vi "select standards.vi"(0 "standards array":T5=[{"Standard Description"="Nitrate (molar)", "standards setup"={"integration time"=0.0, "rinse time"=0.0, "sample time"=0.0, "sample type"=0}, "Standard C"=[0.0, 1e-05, 3e-05, 0.0001, 0.0003, 0.001], "extinction"=array[316 elements], "Your name"="Monroe Weber-Shirk", "correlation coef"=[], "units"=""}, {"Standard Description"="Methylene Blue (molar)", "standards setup"={"integration time"=0.0, "rinse time"=0.0, "sample time"=0.0, "sample type"=0}, "Standard C"=[0.0, 1e-05, 3e-05, 0.0001, 0.0003, 0.001], "extinction"=array[316 elements], "Your name"="Monroe Weber-Shirk", "correlation coef"=[], "units"=""}, {"Standard Description"="Nitrate (molar)", "standards setup"={"integration time"=0.0, "rinse time"=0.0, "sample time"=0.0, "sample type"=0}, "Standard C"=[0.0, 1e-05, 3e-05, 0.0001, 0.0003, 0.001], "extinction"=[6e-05, 0.00221, 0.00306, 0.00317, 0.00265, 0.00207, 0.00119, 0.00025, -0.00096, -0.00199, -0.00326, -0.00411, -0.00514, -0.00601, -0.00637, -0.00648, -0.00656, -0.00639, -0.00598, -0.00572, -0.00506, -0.00451, -0.00396, -0.0035, -0.00303, -0.00267, -0.00244, -0.00225, -0.00195, -0.00143, -0.00079, 3e-05, 0.0008, 0.00166, 0.00238, 0.00297, 0.00341, 0.00378, 0.0039, 0.00392, 0.00384, 0.00372, 0.00352, 0.00314, 0.00282, 0.00242, 0.00177, 0.00137, 0.00077, -1e-05, -0.00059, -0.00108, -0.00134, -0.00131, -0.00105, -0.00088, -0.00057, -0.00032, -0.00022, -0.00033, -0.00038, -0.00019, -0.00021, -0.00013, -0.00021, -0.00012, -0.00018, -6e-05, -0.00015, -0.00013, -7e-05, -1e-05, 4e-05, 0.00028, 0.00035, 0.00048, 0.00077, 0.0008, 0.00097, 0.00123, 0.00125, 0.00146, 0.00151, 0.00158, 0.00175, 0.00189, 0.00192, 0.00209, 0.00259, 0.00344, 0.00344, 0.00314, 0.00273, 0.00338, 0.00329, 0.00483, 0.00416, 0.00453, 0.00415, 0.0057, 0.00456, 0.00387, 0.00733, 0.00433, 0.00578, 0.00793, 0.00433, 0.00503, 0.00907, 0.00512, 0.00527, 0.00619, 0.00883, 0.00532, 0.00614, 0.00546, 0.01057, 0.01022, 0.00575, 0.00856, 0.01062, 0.01115, 0.00621, 0.00558, 0.00915, 0.00848, 0.00535, 0.00787, 0.00842, 0.00877, 0.00704, 0.00596, 0.00531, 0.00262, 0.00599, 0.00656, 0.00518, 0.00746, 0.01216, 0.0121, 0.00685, 0.00506, 0.0082, 0.00939, 0.00521, 0.00415, 0.00613, 0.00923, 0.00846, 0.01092, 0.01307, 0.00959, 0.0108, 0.01184, 0.01274, 0.00772, 0.01136, 0.01332, 0.00874, 0.0079, 0.0115, 0.01463, 0.01071, 0.00805, 0.01184, 0.0133, 0.01077, 0.00883, 0.01077, 0.00929, 0.009, 0.00866, 0.00807, 0.00978, 0.01129, 0.00897, 0.00906, 0.0057, 0.01086, 0.01492, 0.0093, 0.00859, 0.01165, 0.01368, 0.01042, 0.00794, 0.0093, 0.00512, -0.00669, -0.0079, -0.00685, 0.00434, -0.00195, 0.00642, 0.00312, 0.00416, -0.00061, -0.00059, -0.0019, -0.00566, -0.00833, 0.00254, 0.0, -0.00189, 0.00862, 0.00765, 0.00112, -0.00064, 0.0028, 0.00683, 0.00155, -0.0003, 0.0054, 0.00462, -0.00639, 0.00265, 0.00604, -0.00057, -0.00447, 0.00471, -0.00041, -0.01329, -0.00877, -0.0001, 0.0025, -0.01448, -0.01643, -0.01341, -0.0164, -0.00784, 0.00132, -0.00469, -0.00727, -0.00599, -0.00289, -0.0079, -0.00978, -0.00033, -0.0065, -0.01058, 0.00389, 0.00607, -0.00247, 0.00625, 0.00309, 0.0075, 0.00675, 0.00238, 0.02153, 0.00531, 0.00671, 0.01777, 0.00942, 0.01489, 0.02458, 0.00833, 0.00894, 0.0129, 0.01617, 0.02844, 0.01483, 0.01608, 0.02296, 0.01797, 0.01881, 0.0142, 0.00575, 0.00914, 0.01087, 0.01379, 0.01463, 0.0223, 0.00849, 0.01046, 0.00225, 0.01255, 0.00628, 0.00013, -0.01025, -0.00317, -0.00169, -0.00013, 0.014, 0.00627, 0.02648, 0.01156, 0.01533, 0.0162, 0.012, 0.00538, 0.01255, -0.00395, -0.00947, -0.0081, -0.0059, -0.00109, 0.01068, 0.00973, 0.0028, 0.00073, 0.01567, 0.01887, 0.02369, 0.02372, 0.01115, 0.01058, 0.00817, 0.00433, 0.00431, 0.01495, -0.00257, 0.00178, -0.00054, 0.00404, 0.01396, 0.00617], "Your name"="Monroe Weber-Shirk", "correlation coef"=[], "units"=""}] {"correlation coef" format="%.3f"; "extinction" format="%.2e"; "Standard C" format="%^.2e"; "standards setup"."sample type" items=["Sample Cuvet", "Sipper Cell", "No Dialog"]; "standards setup"."sample time" min=0.0 max=100.0 step=1.0 format="%.1f"; "standards setup"."rinse time" min=0.0 max=100.0 step=1.0 format="%.1f"; "standards setup"."integration time" format="%.1f"}, 11 "standard cluster array in":T2 {"Absorbance" format="%.2e"; "Concentrations" format="%.3e"; "Setup"."sample type" items=["Sample Cuvet", "Sipper Cell", "No Dialog"]; "Setup"."sample time" min=0.0 max=100.0 step=1.0 format="%.1f"; "Setup"."rinse time" min=0.0 max=100.0 step=1.0 format="%.1f"; "Setup"."integration time" format="%.1f"}) -> (10 "mixture cluster":T1 {"H array" format="%.2f"}, 15 "standard cluster array out":T2 {"Absorbance" format="%.2e"; "Concentrations" format="%.3e"; "Setup"."sample type" items=["Sample Cuvet", "Sipper Cell", "No Dialog"]; "Setup"."sample time" min=0.0 max=100.0 step=1.0 format="%.1f"; "Setup"."rinse time" min=0.0 max=100.0 step=1.0 format="%.1f"; "Setup"."integration time" format="%.1f"})   [LabVIEW 2015]
uses:
  standards array.ctl
  settings.ctl
  standard cluster array.ctl
  standard cluster.ctl
  mixture cluster.ctl
panel:
  in  "empty standard cluster array":T2 {"Absorbance" format="%.2e"; "Concentrations" format="%.3e"; "Setup"."sample type" items=["Sample Cuvet", "Sipper Cell", "No Dialog"]; "Setup"."sample time" min=0.0 max=100.0 step=1.0 format="%.1f"; "Setup"."rinse time" min=0.0 max=100.0 step=1.0 format="%.1f"; "Setup"."integration time" format="%.1f"}
  in  "empty array":T5 {"correlation coef" format="%.3f"; "extinction" format="%.2e"; "Standard C" format="%^.2e"; "standards setup"."sample type" items=["Sample Cuvet", "Sipper Cell", "No Dialog"]; "standards setup"."sample time" min=0.0 max=100.0 step=1.0 format="%.1f"; "standards setup"."rinse time" min=0.0 max=100.0 step=1.0 format="%.1f"; "standards setup"."integration time" format="%.1f"}
  in  "?":bool
  in  "Standards available":cluster{"description":string, "selected":bool}[](array[cluster])
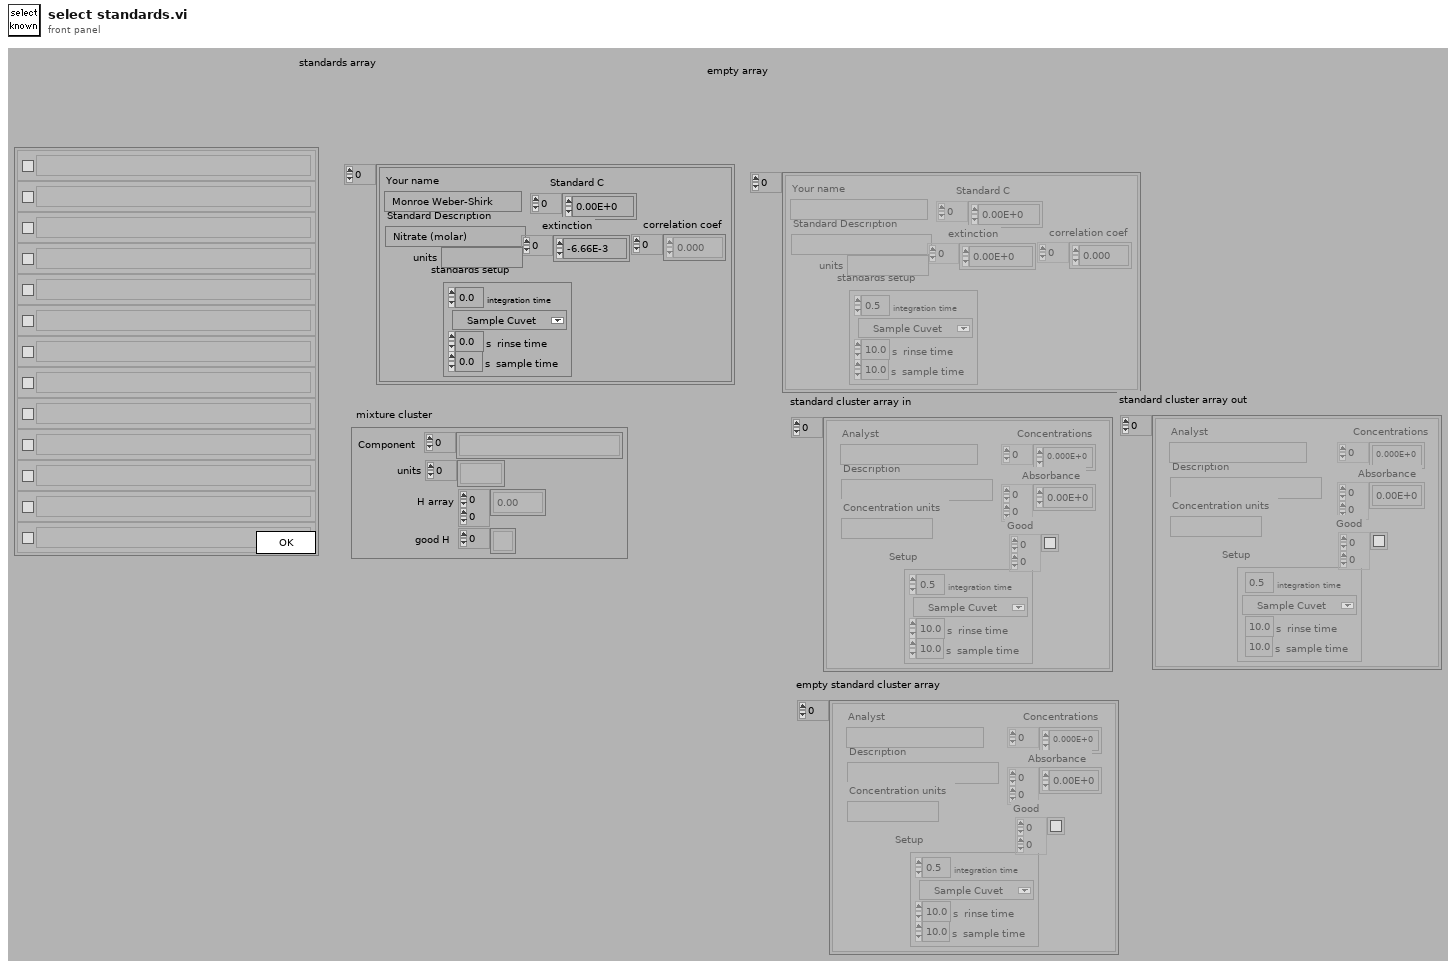
[diagram p1: front panel]
types:
  T1 = typedef "mixture cluster.ctl" = cluster{"Component":string[], "units":string[], "H array":dbl[][], "good H":bool[]}
  T2 = typedef "standard cluster array.ctl" = T3[]
  T3 = typedef "standard cluster.ctl" = cluster{"Description":string, "Setup":T4, "Concentrations":dbl[], "Absorbance":dbl[][], "Analyst":string, "Concentration units":string, "Good":bool[][]}
  T4 = typedef "settings.ctl" = cluster{"integration time":sgl, "rinse time":dbl[unit], "sample time":dbl[unit], "sample type":u16}
  T5 = typedef "standards array.ctl" = cluster{"Standard Description":string, "standards setup":T4, "Standard C":dbl[], "extinction":dbl[], "Your name":string, "correlation coef":dbl[], "units":string}[]
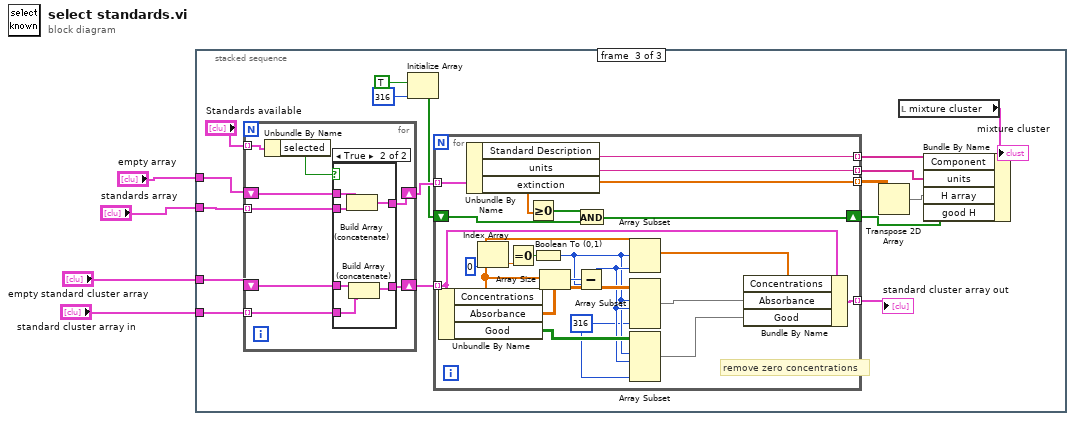
[diagram p0: block diagram]
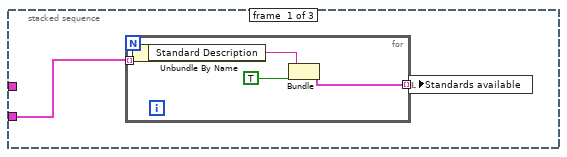
[diagram p2: hidden frame]
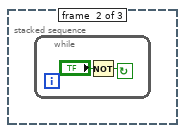
[diagram p3: hidden frame]
diagram:
  n1 = stacked-sequence {
    tunnel: "standards array" -> [w5 _ w29]
    tunnel: "empty array" -> [_ _ w28]
    tunnel: "empty standard cluster array" -> [_ _ w27]
    tunnel: "standard cluster array in" -> [_ _ w26]
    frame #0 {
      n2 = for {
        tunnel: w5 -> [w10] mode=indexing
        tunnel: [w7] -> w6 mode=indexing
        n3 = Unbundle By Name(w10) -> ("Standard Description"=w8:string)
        n4 = Bundle("Standard Description"=w8, TRUE) -> (w7:cluster{"Standard Description":string, bool})  [unwired: 1 in]
      }
      n5 = local write "Standards available"(w6) -> ()
    }
    frame #1 {
      n6 = while {
        stop <- w11 continue-if-true
        n7 = Not(x="?") -> (.not. x?=w11:bool)
      }
    }
    frame #2 {
      n8 = for {
        tunnel: "Standards available" -> [w60] mode=indexing
        tunnel: w29 -> [w58] mode=indexing
        shift-right: [w56] -> w25
        shift-left: w28 -> [w57]
        shift-right: [w55] -> w20
        shift-left: w27 -> [w54]
        tunnel: w26 -> [w53] mode=indexing
        n9 = Unbundle By Name(w60) -> ("selected"=w59:bool)
        n10 = case shown="True" w59 {
          tunnel: w58 -> [_ w68]
          tunnel: w57 -> [w62 w67]
          tunnel: [w62 w66] -> w56
          tunnel: [w61 w64] -> w55
          tunnel: w54 -> [w61 w65]
          tunnel: w53 -> [_ w63]
          frame False {
          }
          frame True {
            n11 = Build Array (concatenate)(w67, w68) -> (w66:T5)
            n12 = Build Array (concatenate)(w65, w63) -> (w64:T2)
          }
        }
      }
      n13 = Initialize Array(TRUE, 316) -> (w22:bool[])
      n14 = for {
        tunnel: w25 -> [w52] mode=indexing
        tunnel: [w51] -> w15 mode=indexing
        tunnel: [w50] -> w14 mode=indexing
        shift-right: [w46] -> w13
        shift-left: w22 -> [w47]
        tunnel: [w49] -> w21 mode=indexing
        tunnel: w20 -> [w45] mode=indexing
        tunnel: [w44] -> w19 mode=indexing
        w34 = 316
        # "remove zero concentrations"
        n15 = Unbundle By Name(w45) -> ("Concentrations"=w40:dbl[], "Absorbance"=w38:dbl[][], "Good"=w37:bool[][])
        n16 = Unbundle By Name(w52) -> ("Standard Description"=w51:string, "units"=w50:string, "extinction"=w49:dbl[])
        n17 = Index Array(array=w40, index=0) -> (element=w42:dbl)
        n18 = Equal To 0?(x=w42) -> (x = 0?=w41:bool)
        n19 = Greater Or Equal To 0?(x=w49) -> (x >= 0?=w48:bool[])
        n20 = Boolean To (0,1)(Boolean=w41) -> (0, 1=w35:i16)
        n21 = Array Size(array=w40) -> (size(s)=w39:i32)
        n22 = Subtract(x=w39, y=w35) -> (x-y=w36:i32)
        n23 = And(x=w48, y=w47) -> (x .and. y?=w46:bool[])
        n24 = Array Subset(array=w40, index=w35, length=w36) -> (w33:dbl[])
        n25 = Array Subset(array=w38, index (row)=w35, length (row)=w36, length (col)=w34) -> (w32:dbl[][])  [unwired: 1 in]
        n26 = Array Subset(array=w37, index (row)=w35, length (row)=w36, length (col)=w34) -> (w31:bool[][])  [unwired: 1 in]
        n27 = Bundle By Name(cluster=w45, "Concentrations"=w33, "Absorbance"=w32, "Good"=w31) -> (w44:T3)
      }
      "standard cluster array out" <- w19
      n28 = Transpose 2D Array(2D array=w21) -> (transposed array=w16:dbl[][])
      n29 = local read "mixture cluster"() -> (w17:T1)
      n30 = Bundle By Name(cluster=w17, "Component"=w15, "units"=w14, "H array"=w16, "good H"=w13) -> (→"mixture cluster":T1)
    }
  }
